vi "DSF.Memory.Buffer.New.vi"(8 "error in (no error)":errorcluster, 10 "id":i32, 11 "size":u64 format="%x bytes") -> (0 "error out":errorcluster, 3 "Buffer out":refnum<class "DSF.Engine.Memory.Buffer.lvclass">)   [LabVIEW 2016, in "DSF.Engine.lvlib" / "DSF.Engine.Memory.Buffer.lvclass"]
uses:
  DSF.Engine.Memory.Buffer.lvclass
  Submodules/Memory Manager/Source/Classes/Pointer.Internal/Memory.Pointer.Internal.lvclass
  C:/Git/SourceTree/DSF/Source/Submodules/Memory Manager/Source/Classes/Pointer.Internal/Memory.Pointer.Internal.lvclass
  C:/Git/SourceTree/DSF/Source/Submodules/Memory Manager/Source/Classes/Pointer/Memory.Pointer.lvclass
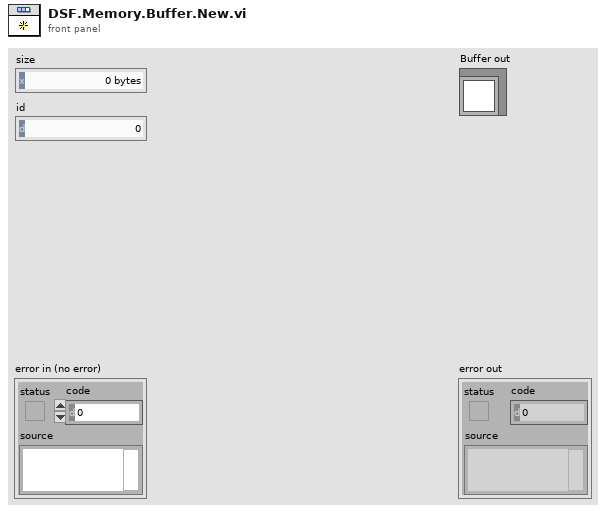
[diagram p1: front panel]
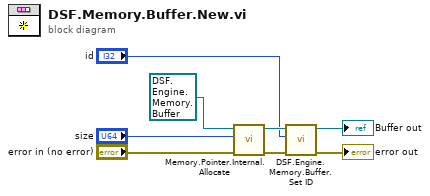
[diagram p0: block diagram]
diagram:
  n1 = call "Memory.Pointer.Internal.Allocate.vi"("error in (no error)"="error in (no error)", "size"="size", "pointer in"=refnum<class "DSF.Engine.Memory.Buffer.lvclass"> refnum ("DSF.Memory.Buffer.lvclass")) -> ("error out"=w6:errorcluster, "pointer out"=w2:refnum<class "DSF.Engine.Memory.Buffer.lvclass">)  [unwired: 7 in]
  n2 = call "DSF.Engine.Memory.Buffer.Set ID.vi"("error in (no error)"=w6, "id"="id", "Buffer in"=w2) -> ("error out"=→"error out":errorcluster, "Buffer out"=→"Buffer out":refnum<class "DSF.Engine.Memory.Buffer.lvclass">)  [unwired: 7 in]
